vi "NI 影像處理二值化、過濾、旋轉.vi"() -> ()   [LabVIEW 2019]
panel:
  in  "stop":bool
  out "Image":T1(plugin-control)
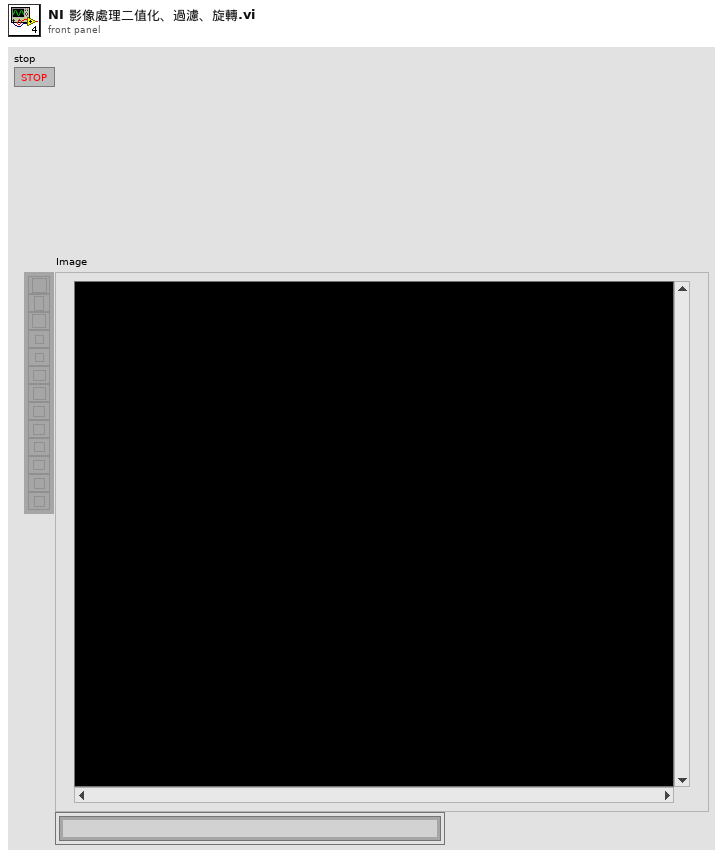
[diagram p1: front panel]
types:
  T1 = typedef "IMAQ Image.ctl" = refnum<image>
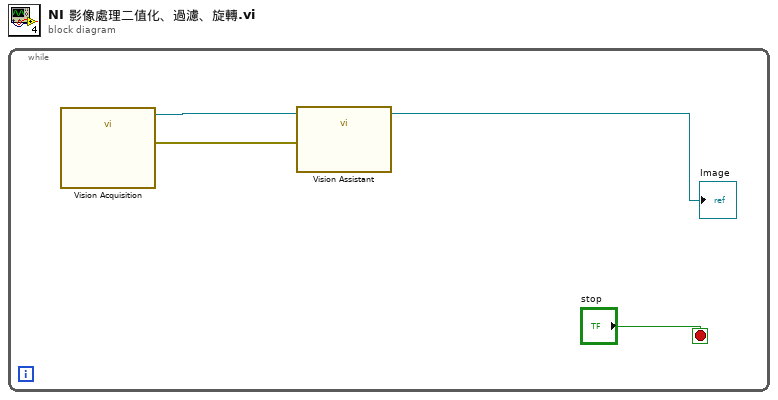
[diagram p0: block diagram]
diagram:
  n1 = while {
    stop <- "stop" stop-if-true
    n2 = call "Vision Acquisition"() -> ("Image Out"=w4:T1, "error out"=w3:errorcluster)  [unwired: 25 in, 1 out]
    n3 = call "Vision Assistant"("Image In"=w4, "error in"=w3) -> ("Image Out"=→"Image":T1)  [unwired: 24 in, 1 out]
  }
